vi "oa_SCL Filter Zero Label.vi"(1 "zero coordinate":i16, 2 "scale specs 2":cluster{"coordinate":i16, "label":string}[](array[cluster])) -> (0 "scale specs":cluster{"coordinate":i16, "label":string}[](array[cluster]))   [LabVIEW 2017]
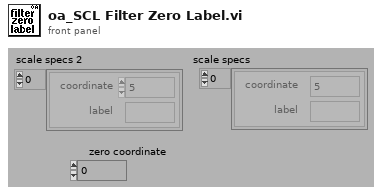
[diagram p1: front panel]
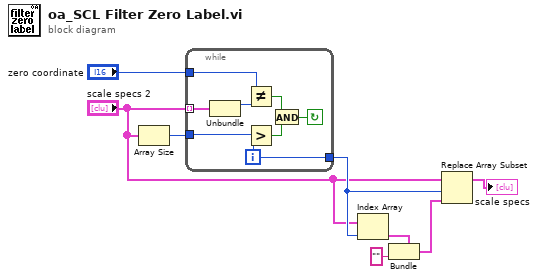
[diagram p0: block diagram]
diagram:
  n1 = Array Size(array="scale specs 2") -> (size(s)=w1:i32)
  n2 = while {
    tunnel: w1 -> [w12]
    tunnel: [w13] -> w3
    tunnel: "zero coordinate" -> [w14]
    tunnel: "scale specs 2" -> [w16] mode=indexing
    i -> [w13]
    stop <- w9 continue-if-true
    n3 = Unbundle(w16) -> ("coordinate"=w15:i16)  [unwired: 1 out]
    n4 = Not Equal?(x=w14, y=w15) -> (x != y?=w11:bool)
    n5 = Greater?(x=w12, y=w13) -> (0:w10:bool)
    n6 = And(x=w11, y=w10) -> (x .and. y?=w9:bool)
  }
  n7 = Index Array(array="scale specs 2", index=w3) -> (element=w7:cluster{"coordinate":i16, "label":string})
  n8 = Bundle(cluster=w7, "label"="") -> (w5:cluster{"coordinate":i16, "label":string})  [unwired: 1 in]
  n9 = Replace Array Subset(array="scale specs 2", new element=w5, index=w3) -> (→"scale specs":cluster{"coordinate":i16, "label":string}[])
